vi "holdPosition.vi"(8 "BL":dbl, 9 "BR":dbl, 10 "FL":dbl, 11 "FR":dbl) -> ()   [LabVIEW 2020]
uses:
  <vilib>/Rock Robotics/WPI/ThirdParty/REV Robotics/REVLib/Typedef/Spark MAX Control Type.ctl
  Robot Global Data.vi
  <vilib>/addons/control/pid/pid.llb/PID (DBL).vi
  <vilib>/addons/control/pid/NI_PID_pid.lvlib
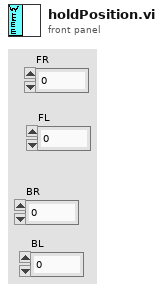
[diagram p1: front panel]
types:
  T1 = typedef "Spark MAX Control Type.ctl" = enum16{"Percent VBus", "Voltage", "Velocity", "Position", "Smart Motion", "Current", "Smart Velocity"}
  T2 = cluster{"FL":cluster{"proportional gain (Kc)":dbl, "integral time (Ti, min)":dbl, "derivative time (Td, min)":dbl}, "FR":cluster{"proportional gain (Kc)":dbl, "integral time (Ti, min)":dbl, "derivative time (Td, min)":dbl}, "BL":cluster{"proportional gain (Kc)":dbl, "integral time (Ti, min)":dbl, "derivative time (Td, min)":dbl}, "BR":cluster{"proportional gain (Kc)":dbl, "integral time (Ti, min)":dbl, "derivative time (Td, min)":dbl}}
  T3 = typedef "WPI_MotorControlDeviceRef.ctl" = cluster{"DeviceStatus":errorcluster, "Type":T4, "PWM":cluster{"PWM Channel":T5, "DeadBand":T6}, "CAN":cluster{"Device Number":u8, "SetOutput VI Ref":variant, "GetOutput VI Ref":variant, "Enable VI Ref":variant, "Disable VI Ref":variant, "Data":variant}, "Invert":bool, "DIO PWM":cluster{"PWM \"Enable\" Channel":T5, "DIOChannel":T7, "PWM Rate":dbl}}
  T4 = typedef "WPI_MotorControlType.ctl" = enum16{"PWM", "CAN", "DIO PWM"}
  T5 = typedef "FPGA_DIOPWMChannel.ctl" = enum8{"PWM 0", "PWM 1", "PWM 2", "PWM 3", "PWM 4", "PWM 5", "PWM 6", "PWM 7", "PWM 8", "PWM 9", "PWM MXP 0", "PWM MXP 1", "PWM MXP 2", "PWM MXP 3", "PWM MXP 4", "PWM MXP 5", "PWM MXP 6", "PWM MXP 7", "PWM MXP 8", "PWM MXP 9", "Invalid"}
  T6 = typedef "WPI_PWMDeadband.ctl" = cluster{"Name":string, "maxPositivePwm":i32, "minPositivePwm":i32, "centerPwm":i32, "maxNegativePwm":i32, "minNegativePwm":i32, "angularRange":u16}
  T7 = typedef "FPGA_DIOChannel.ctl" = enum8{"DIO 0", "DIO 1", "DIO 2", "DIO 3", "DIO 4", "DIO 5", "DIO 6", "DIO 7", "DIO 8", "DIO 9", "DIO MXP 0", "DIO MXP 1", "DIO MXP 2", "DIO MXP 3", "DIO MXP 4", "DIO MXP 5", "DIO MXP 6", "DIO MXP 7", "DIO MXP 8", "DIO MXP 9", "DIO MXP 10", "DIO MXP 11", "DIO MXP 12", "DIO MXP 13", "DIO MXP 14", "DIO MXP 15", "SPI Port CS1", "SPI Port CS2", "SPI Port CS3", "SPI Port MISO", "SPI Port MOSI", "Invalid"}
  T8 = cluster{"proportional gain (Kc)":dbl, "integral time (Ti, min)":dbl, "derivative time (Td, min)":dbl}
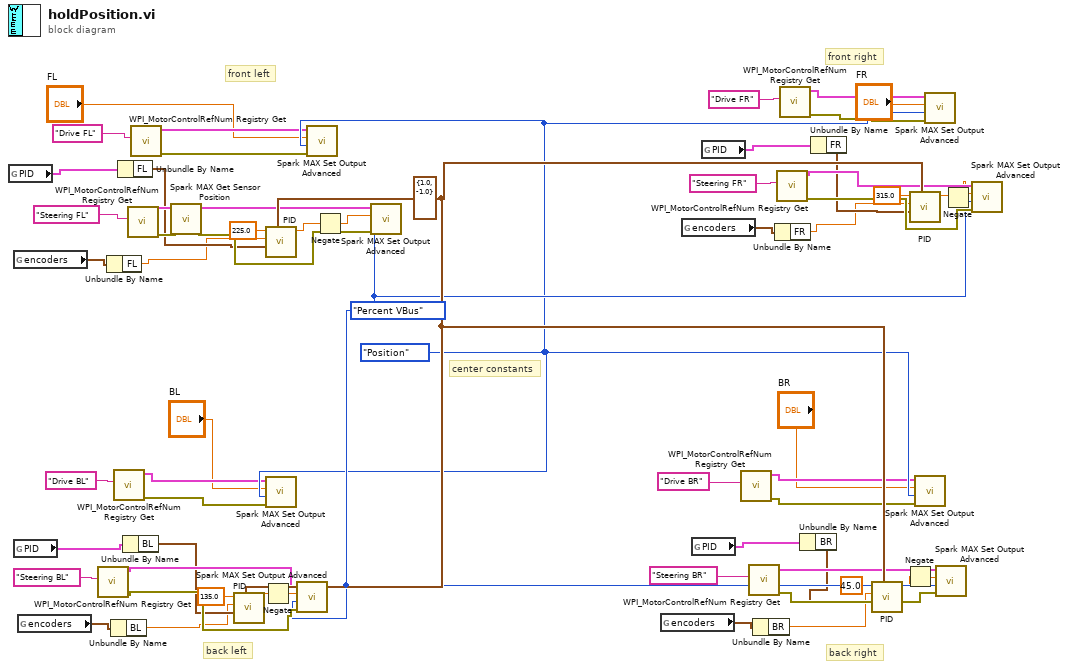
[diagram p0: block diagram]
diagram:
  w41 = Spark_MAX_Control_Type."Position" ("Control Mode")
  w42 = Spark_MAX_Control_Type."Percent VBus" ("Control Mode")
  w51 = cluster{"output high":dbl, "output low":dbl} {"output high"=1.0, "output low"=-1.0} ("output range")
  # "center constants"
  # "back right"
  # "back left"
  # "front right"
  # "front left"
  n1 = global read "Robot Global Data.vi" "PID"() -> (w22:T2)
  n2 = global read "Robot Global Data.vi" "encoders"() -> (w8:cluster{"FL":dbl, "FR":dbl, "BL":dbl, "BR":dbl})
  n3 = global read "Robot Global Data.vi" "PID"() -> (w24:T2)
  n4 = global read "Robot Global Data.vi" "encoders"() -> (w2:cluster{"FL":dbl, "FR":dbl, "BL":dbl, "BR":dbl})
  n5 = call <vilib>:"WPI_MotorControlRefNum Registry Get.vi"("refnum name"="Steering BL") -> ("error out"=w45:errorcluster, "MotorControlDevRef"=w46:T3)  [unwired: 9 in]
  n6 = Unbundle By Name(w8) -> ("FL"=w7:dbl)
  n7 = Unbundle By Name(w2) -> ("BL"=w1:dbl)
  n8 = call <vilib>:"WPI_MotorControlRefNum Registry Get.vi"("refnum name"="Drive BL") -> ("error out"=w39:errorcluster, "MotorControlDevRef"=w40:T3)  [unwired: 9 in]
  n9 = Unbundle By Name(w22) -> ("FL"=w21:T8)
  n10 = Unbundle By Name(w24) -> ("BL"=w23:T8)
  n11 = call <vilib>:"WPI_MotorControlRefNum Registry Get.vi"("refnum name"="Steering FL") -> ("error out"=w57:errorcluster, "MotorControlDevRef"=w56:T3)  [unwired: 9 in]
  n12 = call <vilib>:"WPI_MotorControlRefNum Registry Get.vi"("refnum name"="Drive FL") -> ("error out"=w37:errorcluster, "MotorControlDevRef"=w38:T3)  [unwired: 9 in]
  n13 = call <vilib>:"Spark MAX Get Sensor Position.vi"("error in (no error)"=w57, "MotorControlDevRef in"=w56) -> ("error out"=w49:errorcluster, "MotorControlDevRef out"=w50:T3)  [unwired: 6 in, 2 out]
  n14 = call-poly <vilib>:"PID.vi"("output range"=w51, "PID gains"=w23, "process variable"=w1, "setpoint"=135.0) -> ("output"=w11:dbl)  [unwired: 6 in, 1 out]
  n15 = Negate(x=w11) -> (-x=w12:dbl)
  n16 = call-poly <vilib>:"PID.vi"("output range"=w51, "PID gains"=w21, "process variable"=w7, "setpoint"=225.0) -> ("output"=w16:dbl)  [unwired: 6 in, 1 out]
  n17 = call <vilib>:"Spark MAX Set Output Advanced.vi"("error in (no error)"=w39, "Control Mode"=w41, "Setpoint"="BL", "MotorControlDevRef"=w40) -> ()  [unwired: 6 in, 2 out]
  n18 = call <vilib>:"Spark MAX Set Output Advanced.vi"("error in (no error)"=w45, "Control Mode"=w42, "Setpoint"=w12, "MotorControlDevRef"=w46) -> ()  [unwired: 6 in, 2 out]
  n19 = call <vilib>:"Spark MAX Set Output Advanced.vi"("error in (no error)"=w37, "Control Mode"=w41, "Setpoint"="FL", "MotorControlDevRef"=w38) -> ()  [unwired: 6 in, 2 out]
  n20 = Negate(x=w16) -> (-x=w15:dbl)
  n21 = call <vilib>:"Spark MAX Set Output Advanced.vi"("error in (no error)"=w49, "Control Mode"=w42, "Setpoint"=w15, "MotorControlDevRef"=w50) -> ()  [unwired: 6 in, 2 out]
  n22 = global read "Robot Global Data.vi" "encoders"() -> (w4:cluster{"FL":dbl, "FR":dbl, "BL":dbl, "BR":dbl})
  n23 = global read "Robot Global Data.vi" "encoders"() -> (w6:cluster{"FL":dbl, "FR":dbl, "BL":dbl, "BR":dbl})
  n24 = global read "Robot Global Data.vi" "PID"() -> (w18:T2)
  n25 = global read "Robot Global Data.vi" "PID"() -> (w20:T2)
  n26 = call <vilib>:"WPI_MotorControlRefNum Registry Get.vi"("refnum name"="Drive BR") -> ("error out"=w30:errorcluster, "MotorControlDevRef"=w34:T3)  [unwired: 9 in]
  n27 = call <vilib>:"WPI_MotorControlRefNum Registry Get.vi"("refnum name"="Steering BR") -> ("error out"=w43:errorcluster, "MotorControlDevRef"=w44:T3)  [unwired: 9 in]
  n28 = Unbundle By Name(w4) -> ("BR"=w3:dbl)
  n29 = Unbundle By Name(w6) -> ("FR"=w5:dbl)
  n30 = call <vilib>:"WPI_MotorControlRefNum Registry Get.vi"("refnum name"="Steering FR") -> ("error out"=w47:errorcluster, "MotorControlDevRef"=w48:T3)  [unwired: 9 in]
  n31 = call <vilib>:"WPI_MotorControlRefNum Registry Get.vi"("refnum name"="Drive FR") -> ("error out"=w35:errorcluster, "MotorControlDevRef"=w36:T3)  [unwired: 9 in]
  n32 = Unbundle By Name(w18) -> ("BR"=w17:T8)
  n33 = Unbundle By Name(w20) -> ("FR"=w19:T8)
  n34 = call-poly <vilib>:"PID.vi"("output range"=w51, "PID gains"=w17, "process variable"=w3, "setpoint"=45.0) -> ("output"=w10:dbl)  [unwired: 6 in, 1 out]
  n35 = Negate(x=w10) -> (-x=w9:dbl)
  n36 = call-poly <vilib>:"PID.vi"("output range"=w51, "PID gains"=w19, "process variable"=w5, "setpoint"=315.0) -> ("output"=w14:dbl)  [unwired: 6 in, 1 out]
  n37 = call <vilib>:"Spark MAX Set Output Advanced.vi"("error in (no error)"=w30, "Control Mode"=w41, "Setpoint"="BR", "MotorControlDevRef"=w34) -> ()  [unwired: 6 in, 2 out]
  n38 = call <vilib>:"Spark MAX Set Output Advanced.vi"("error in (no error)"=w35, "Control Mode"=w41, "Setpoint"="FR", "MotorControlDevRef"=w36) -> ()  [unwired: 6 in, 2 out]
  n39 = call <vilib>:"Spark MAX Set Output Advanced.vi"("error in (no error)"=w43, "Control Mode"=w42, "Setpoint"=w9, "MotorControlDevRef"=w44) -> ()  [unwired: 6 in, 2 out]
  n40 = Negate(x=w14) -> (-x=w13:dbl)
  n41 = call <vilib>:"Spark MAX Set Output Advanced.vi"("error in (no error)"=w47, "Control Mode"=w42, "Setpoint"=w13, "MotorControlDevRef"=w48) -> ()  [unwired: 6 in, 2 out]
